vi "Read async.vi"(8 "error in":errorcluster, 11 "module editor node in":refnum<class "module editor node.lvclass">) -> (0 "error out":errorcluster, 2 "async module":refnum<class "asynchronous execution module configuration.lvclass">, 3 "module editor node out":refnum<class "module editor node.lvclass">)   [LabVIEW 2013, in "PL Framework Configuration Tool.lvlib" / "module editor node.lvclass"]
uses:
  module editor node.lvclass
  asynchronous execution module/configuration/asynchronous execution module configuration.lvclass
  module editor node.lvclass/module editor node.ctl
  <vilib>/NI/Tag Bus Module Framework/root configuration/TBM configuration.lvclass/TBM configuration.ctl
  <vilib>/NI/Tag Bus Module Framework/root configuration/create GUID.vi
  <vilib>/NI/Tag Bus Module Framework/root configuration/TBM configuration.lvclass
panel:
  out "instance ID":string
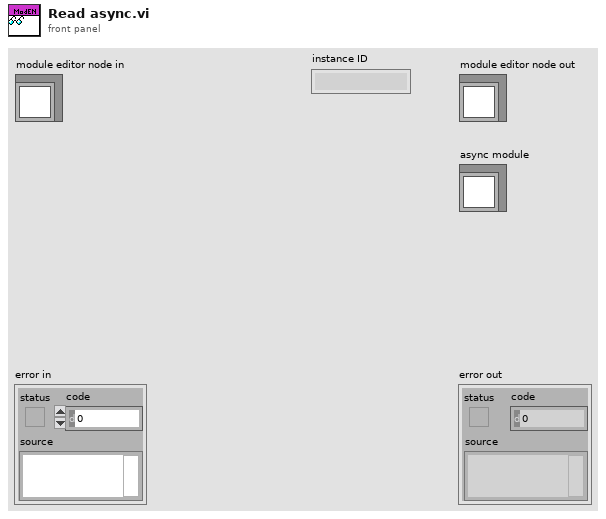
[diagram p1: front panel]
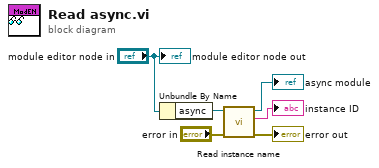
[diagram p0: block diagram]
diagram:
  n1 = Unbundle By Name("module editor node in") -> ("async"=w4:refnum<class "asynchronous execution module configuration.lvclass">)
  n2 = call <vilib>:"Read instance name.vi"("error in"="error in", "configuration in"=w4) -> ("error out"=→"error out":errorcluster, "instance id"=→"instance ID":string, "configuration out"=→"async module":refnum<class "asynchronous execution module configuration.lvclass">)  [unwired: 7 in]
  "module editor node out" <- "module editor node in"
